vi "tasklist_kill.vi"(8 "error in (no error)":errorcluster, 11 "pid":i32=-1) -> (0 "error out":errorcluster)   [LabVIEW 2015, in "lv-bin-windows.lvlib" / "v1.lvlib"]
uses:
  v1.lvlib
  <userlib>/antonio-alexander/lv-bin/lv-bin/public/api/v1/v1.lvlib
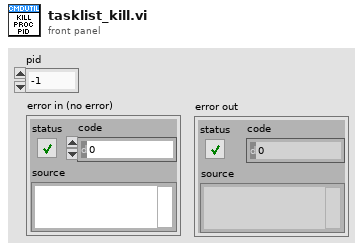
[diagram p1: front panel]
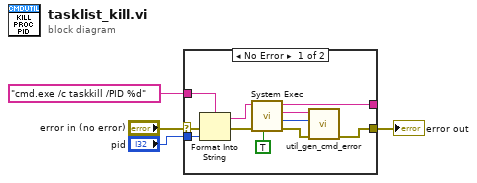
[diagram p0: block diagram]
diagram:
  n1 = case shown="No Error" "error in (no error)" {
    selector: "error in (no error)" -> [w11 w16]
    tunnel: "pid" -> [w13 _]
    tunnel: [w8 w16] -> w3
    tunnel: "cmd.exe /c taskkill /PID %d" ("command line") -> [w10 _]
    tunnel: [w7 _] -> _
    frame No Error {
      n2 = Format Into String(format string=w10, error in=w11, w13) -> (resulting string=w14:string, error out=w12:errorcluster)  [unwired: 1 in]
      n3 = call <vilib>:"System Exec.vi"("run minimized? (F)"=TRUE, "error in (no error)"=w12, "command line"=w14) -> ("error out"=w9:errorcluster, "return code"=w5:i32, "standard error"=w6:string, "standard output"=w7:string)  [unwired: 5 in]
      n4 = call <userlib>:"util_gen_cmd_error.vi"("error in (no error)"=w9, "return_code"=w5, "standard_error"=w6) -> ("error out"=w8:errorcluster)  [unwired: 8 in]
    }
    frame Error {
    }
  }
  "error out" <- w3
